vi "SET_Data.vi"(8 "error in (no error)":errorcluster, 10 "Data":variant, 11 "FakedArray in":refnum<class "FakedArray.lvclass">) -> (0 "error out":errorcluster, 3 "FakedArray out":refnum<class "FakedArray.lvclass">)   [LabVIEW 2021, in "FakedArray.lvclass"]
uses:
  <resource>/plugins/NIIconEditor/Class/FakedArray/FakedArray.lvclass
  <resource>/plugins/NIIconEditor/Class/FakedArray/FakedArray.lvclass/FakedArray.ctl
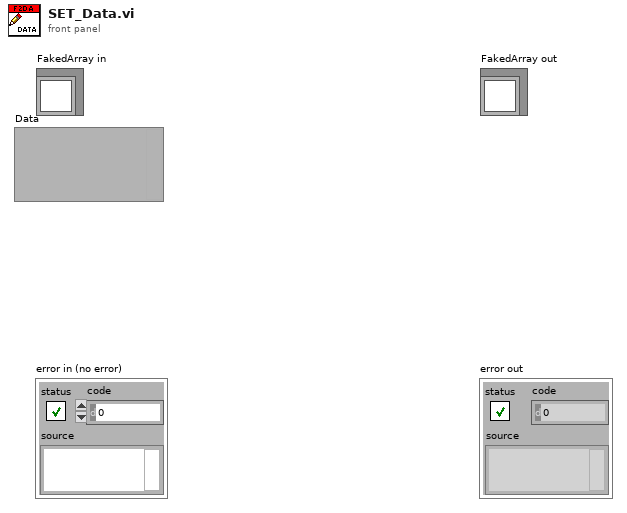
[diagram p1: front panel]
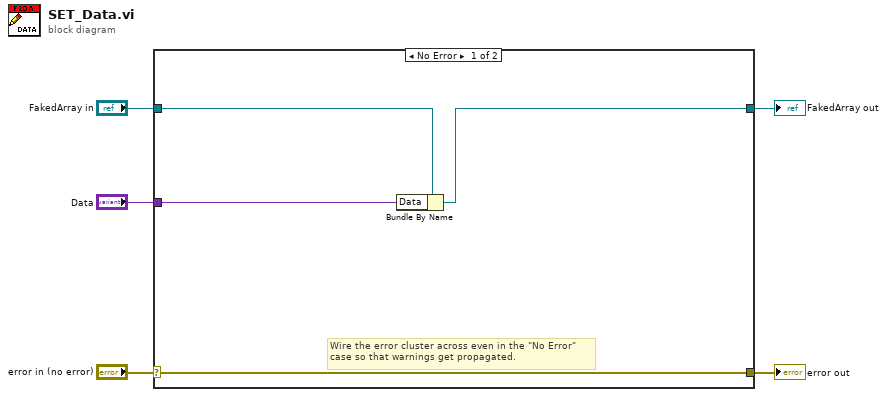
[diagram p0: block diagram]
diagram:
  n1 = case shown="No Error" "error in (no error)" {
    selector: "error in (no error)" -> [w8 w11]
    tunnel: [w8 w11] -> w4
    tunnel: [w7 w10] -> w2
    tunnel: "FakedArray in" -> [w9 w10]
    tunnel: "Data" -> [w6 _]
    frame No Error {
      # "Wire the error cluster across even in the \"No Error\"\ncase so that warnings get propagated."
      n2 = Bundle By Name(cluster=w9, "Data"=w6) -> (w7:refnum<class "FakedArray.lvclass">)
    }
    frame Error {
    }
  }
  "error out" <- w4
  "FakedArray out" <- w2
